vi "play_auto_id-old.vi"(8 "error in":errorcluster, 11 "Swept-Sines-Control-Settings":cluster{"u-max":sgl, "offset":sgl, "Ki":sgl}={"u-max"=1.0, "offset"=0.3, "Ki"=0.0}) -> (0 "error out":errorcluster, 1 "Is-Totally-Stable":bool)   [LabVIEW 2017]
uses:
  controls/SS_SweptSines.ctl
  controls/SS_sin_params.ctl
  controls/SS_input_data_json.ctl
  controls/fit_sos_results.ctl
  controls/auto_id_result.ctl
  controls/SOS_frf_data.ctl
  controls/SS_figures.ctl
  controls/bode_figure.ctl
  controls/logging_selection.ctl
  <vilib>/Utility/error.llb/DialogType.ctl
  <vilib>/FPGAPlugInAG/cRIO-9082/niLvFpga_Open_cRIO-9082.vi
  <vilib>/rvi/interface/common/dynamic/niFpgaDynamicAddResources.vi
  <vilib>/FPGAPlugInAG/Dynamic/niLvFpga_Reset_Dynamic.vi
  <vilib>/rvi/interface/common/niFpgaWaitOnOcc.vi
  <vilib>/Utility/error.llb/Error Cluster From Error Code.vi
  <vilib>/rvi/errors/niLvFpgaAdjustHostInterfaceError.vi
  <vilib>/FPGAPlugInAG/Dynamic/niLvFpga_Run_Dynamic.vi
  <vilib>/FPGAPlugInAG/Dynamic/niLvFpga_Close_Dynamic.vi
  <vilib>/rvi/interface/nirviOpenFPGA/nirviOpenFPGA.xnode
  FPGA Bitfiles/afmimagingcontro_FPGATargetSPARTA_SSfpgasweptsines_lpZqvyn1KNg.lvbitx
  <vilib>/rvi/interface/nirviMethod/nirviMethod.xnode
  <vilib>/rvi/interface/nirviReadWriteControl/nirviReadWriteControl.xnode
  <vilib>/rvi/interface/nirviCloseFPGA/nirviCloseFPGA.xnode
  labview/utils_lib/utils.lvlib
  NiFpgaLv.dll
  <vilib>/rvi/interface/Simulation/niFpgaSimulationCallBeginRW.vi
  <vilib>/addons/_JKI.lib/Serialization/JSON/JKI JSON Serialization.lvlib
  <vilib>/FPGAPlugInAG/Dynamic/niLvFpga_ConfigureFifo_Dynamic.vi
  <vilib>/rvi/errors/niLvFpgaMergeErrorWithErrorCode.vi
panel:
  in  "Tab Control":enum32{"Page 1", "debug"}(tab)
  in  "control-xy-to-zero":bool=TRUE
  in  "Amplitude":dbl=0.12 format="%#_13g"
  in  "ABORT":bool
  out "auto_id_result":T1
  out "fit_sos_result":T3
  in  "theta0":dbl[](array[numeric])=[0.6786, -1.9959, 0.99891, -1.996142, 0.9989]
  out "theta-fit":dbl[](array[numeric])
  out "Bode amplitude":cluster{"W":dbl[], "Magnitude":dbl[]}[](graph) caption="Magnitude Graph"
  in  "Input File (json)":path=path "Z:/afm-cs/sysID/z-axis_sines_info_quick_firstRes.json"
  in  "output-file":path=path "C:/Users/arnold/Documents/afm-cs/labview/first_res_fit.json"
  out "boolean  indicators":T4
  out "Freqs Done":i32(slide) scale=0.0..50.0
  out "number_of_freqs":i32
  out "freq_adjusted":dbl
  in  "SweptSines (in)":T5={"Log-Channel_select"=[FALSE, FALSE, FALSE, FALSE, FALSE, FALSE], "JSON Header"="", "SS-Params-Array"=[], "input_frequency_definitions"={"Amp"=0.0, "Ts"=0.0, "num_periodsMT"=[], "freqs_Hz"=[], "numAve_s"=[], "Nsamp_total"=[], "Nsettle_s"=[], "Ncollect_s"=[]}, "DAC-ADC primary 2"=0, "Channel-Names"=[], "num_chan"=0, "num-freqs"=0, "Input File (json)"=path "Z:/afm-cs/sysID/x-axis_sines_info_intsamps_quick.json"} {"DAC-ADC primary 2" items=["DAC0/ADC0", "DAC1/ADC1", "DAC2/ADC2", "DAC3/ADC3", ""]}
  out "TsTicks":u32
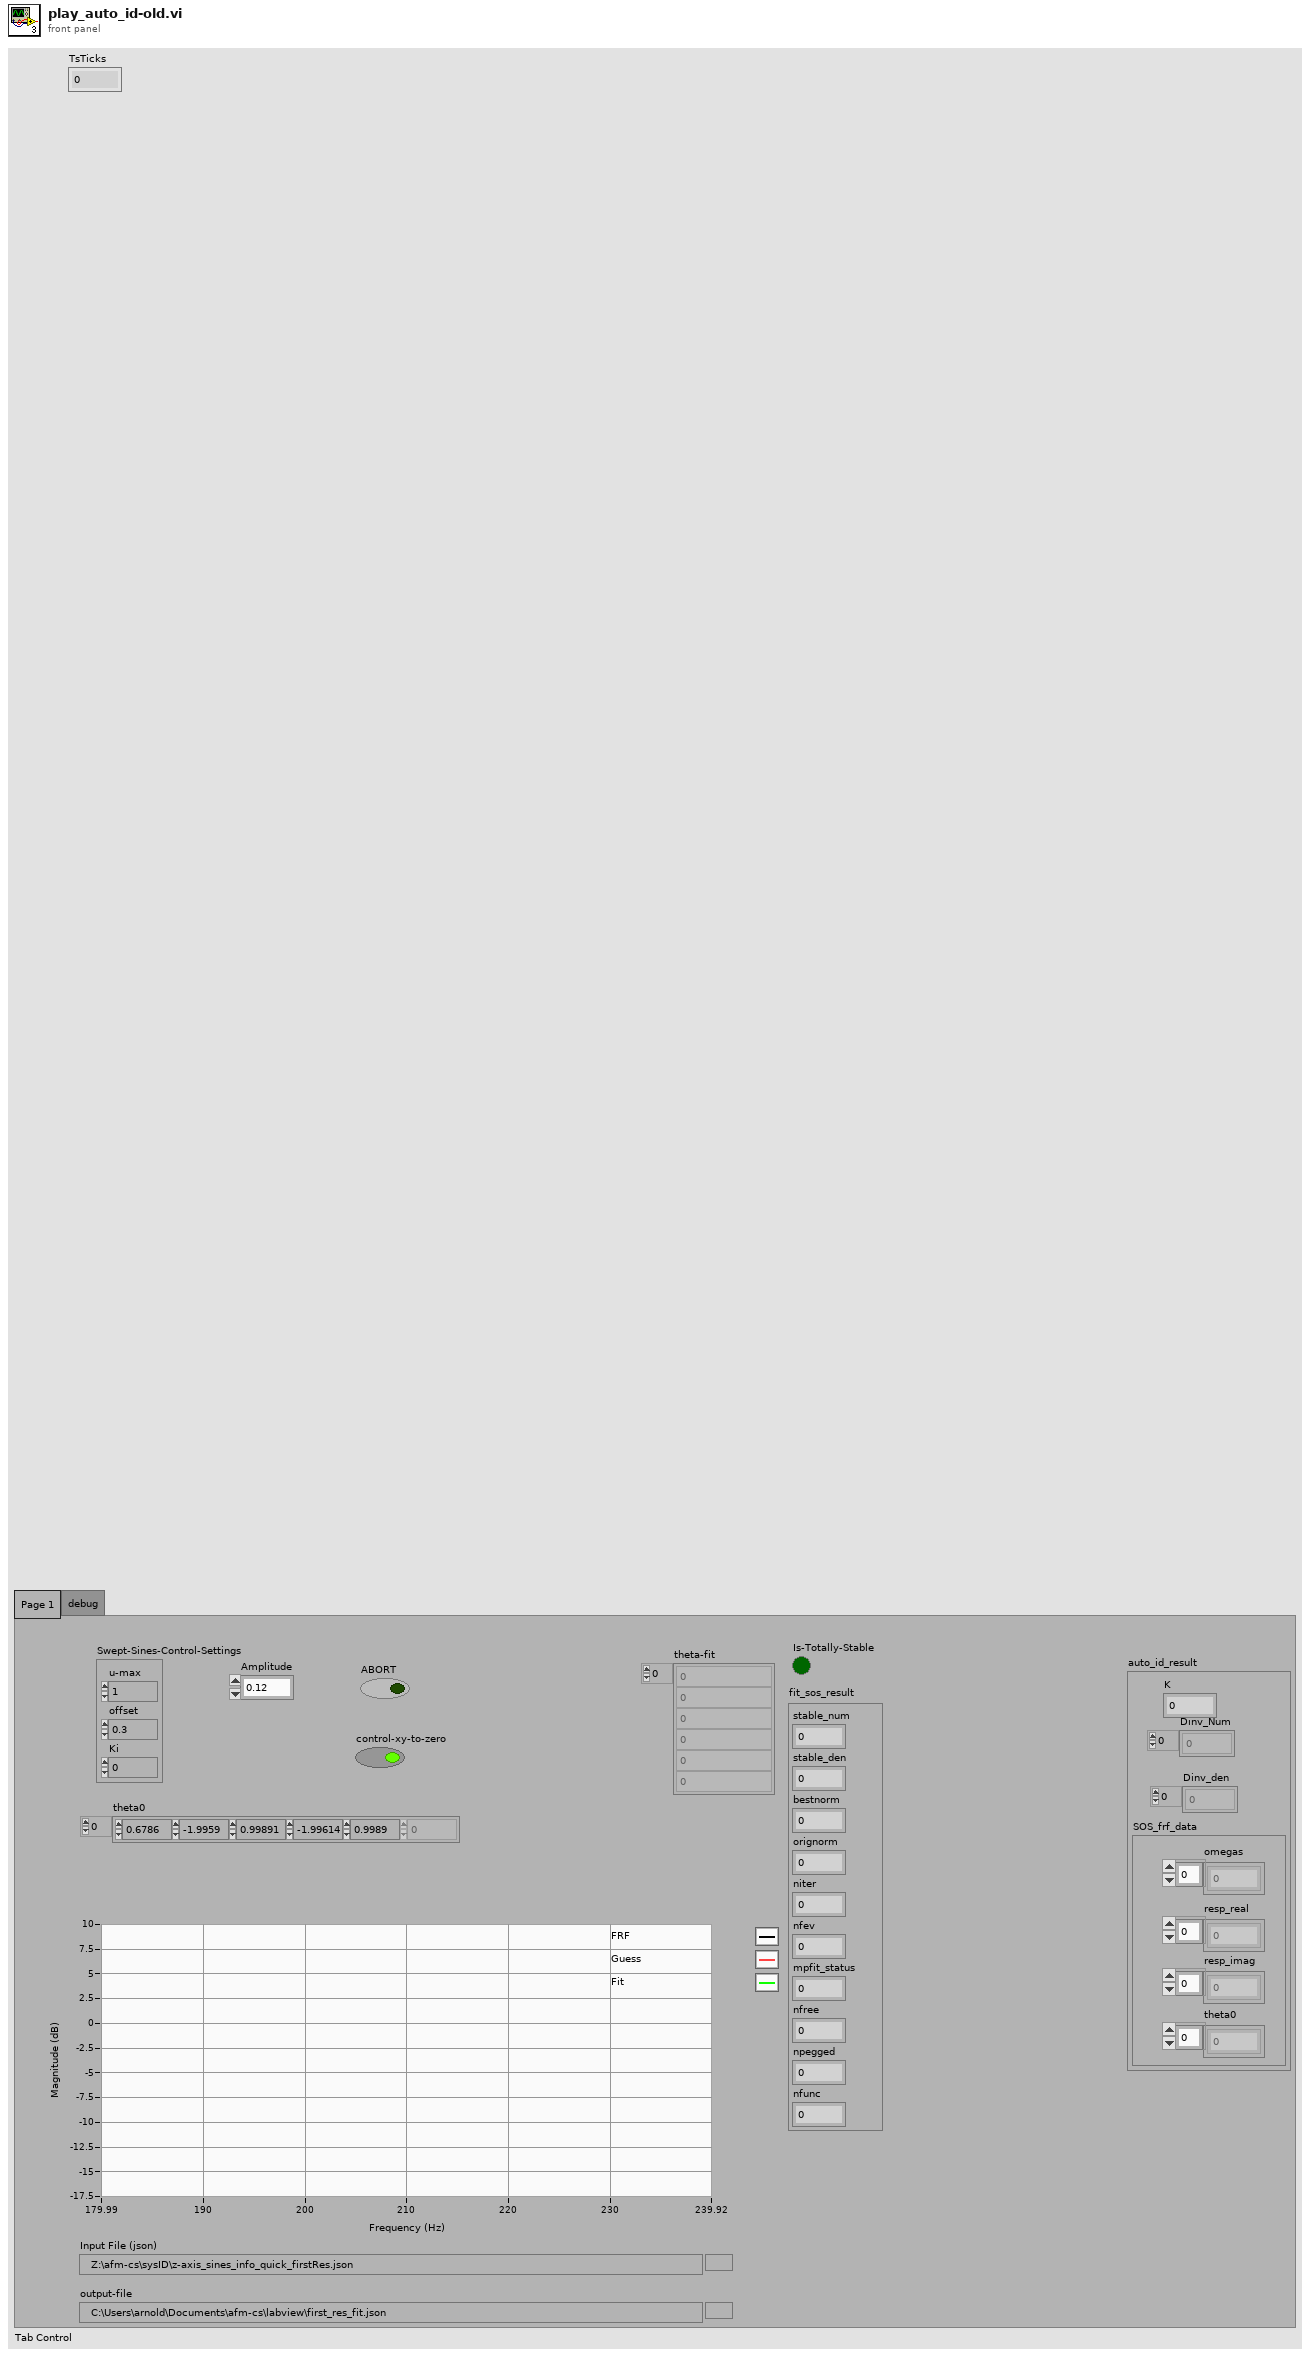
[diagram p1: front panel]
types:
  T1 = typedef "auto_id_result.ctl" = cluster{"Dinv_Num":dbl[], "SOS_frf_data":T2, "Dinv_den":dbl[], "K":dbl}
  T2 = typedef "SOS_frf_data.ctl" = cluster{"omegas":dbl[], "resp_real":dbl[], "resp_imag":dbl[], "theta0":dbl[]}
  T3 = typedef "fit_sos_results.ctl" = cluster{"stable_num":i32, "stable_den":i32, "bestnorm":dbl, "orignorm":dbl, "niter":i32, "nfev":i32, "mpfit_status":i32, "nfree":i32, "npegged":i32, "nfunc":i32}
  T4 = cluster{"unstable-z-traj":bool, "input fifo time-out":bool, "logging fifo timeout":bool, "scanning finished":bool, "unstable-x-traj":bool, "unstable-y-traj":bool, "ABORT":bool, "All Measurements Done":bool, "fpga_finished":bool, "current_scan_finished":bool}
  T5 = typedef "SS_SweptSines.ctl" = cluster{"Log-Channel_select":bool[], "JSON Header":string, "SS-Params-Array":T6[], "input_frequency_definitions":T7, "DAC-ADC primary 2":i16, "Channel-Names":string[], "num_chan":i32, "num-freqs":i32, "Input File (json)":path}
  T6 = typedef "SS_sin_params.ctl" = cluster{"freq":dbl, "num_samples":i32, "Amp":dbl, "Ts":dbl, "N_settle":u32, "Ncollect":i32, "num_periodsMT":i32, "num_averages":i32}
  T7 = typedef "SS_input_data_json.ctl" = cluster{"Amp":dbl, "Ts":dbl, "num_periodsMT":u32[], "freqs_Hz":dbl[], "numAve_s":i32[], "Nsamp_total":u32[], "Nsettle_s":u32[], "Ncollect_s":u32[]}
  T8 = typedef "logging_selection.ctl" = cluster{"Collect reference":bool, "Collect DAC control":bool, "Collect AI-0":bool, "Collect AI-1":bool, "Collect AI-2":bool, "Collect AI-3":bool}
  T9 = typedef "SS_figures.ctl" = cluster{"bode figures":T10, "Freqs Done":refnum<vi>}
  T10 = typedef "bode_figure.ctl" = cluster{"Bode phase":refnum<vi>, "Bode amplitude":refnum<vi>}
  T11 = typedef "FrdData.ctl" = cluster{"Frequency Unit":enum16{"Hz", "rad/s"}, "W":dbl[], "MagDB":dbl[], "PhaseDeg":dbl[], "Resp":cdb[], "Data-name":string}
  T12 = typedef "DialogType.ctl" = u16
  T13 = typedef "SS_experimental-data.ctl" = cluster{"sin-data-out":dbl[][], "Fourier Data":T14, "freq_adjusted?":dbl, "below-nyquist":bool}
  T14 = typedef "SS_FourierData.ctl" = cluster{"E_s":dbl[], "Fourier Coefs":cdb[], "freq-adjusted":dbl}
  T15 = enum16{"open", "replace", "create", "open or create", "replace or create", "replace or create with confirmation"}
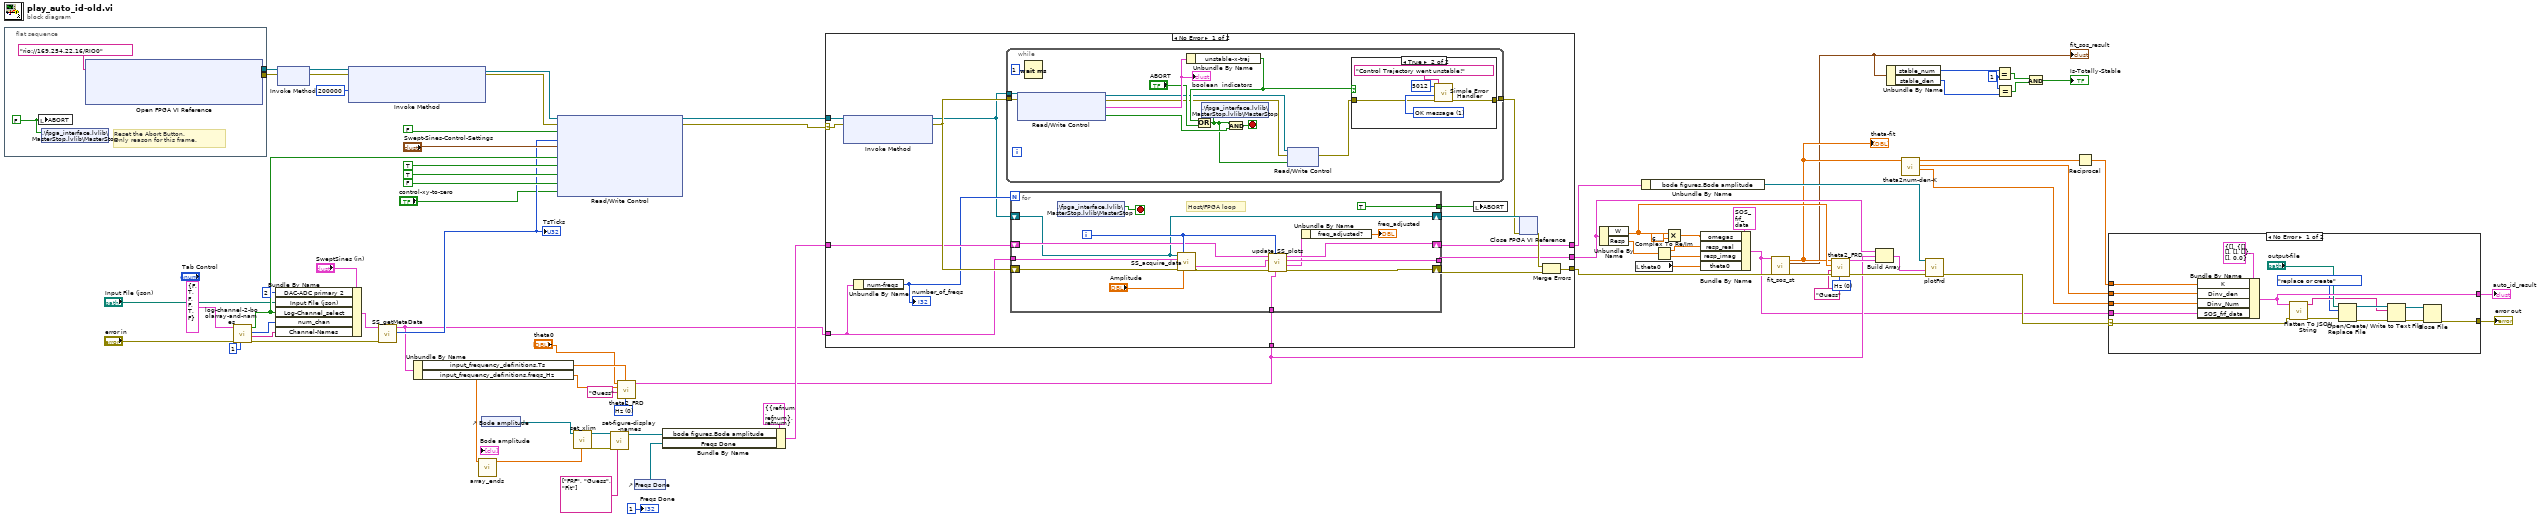
[diagram p0: block diagram]
diagram:
  w14 = 1
  w39 = u16 0 items=["Hz", "rad/s"] ("freq unit")
  w48 = u16 0 items=["Hz", "rad/s"] ("freq unit")
  n1 = flat-sequence {
    tunnel: [w81] -> w77
    tunnel: [w80] -> w76
    frame #0 {
      w79 = FALSE
      # "Reset the Abort Button.\nOnly reason for this frame."
      n2 = local write "ABORT"(w79) -> ()
      n3 = shared-variable ".\\fpga_interface.lvlib\\MasterStop.lvlib\\MasterStop"(w79) -> ()  [unwired: 1 in, 1 out]
      n4 = xnode "Open FPGA VI Reference"("resource name"=tag "rio://169.254.22.16/RIO0") -> ("FPGA VI Reference Out"=w81:refnum<k20>, "error out"=w80:errorcluster)  [unwired: 1 in]
    }
  }
  n5 = call "log-channel-2-boolarray-and-names.vi"("min_number_chan"=i16 1, "error in"="error in", "Logging selection"=T8 {"Collect reference"=FALSE, "Collect DAC control"=TRUE, "Collect AI-0"=FALSE, "Collect AI-1"=FALSE, "Collect AI-2"=TRUE, "Collect AI-3"=FALSE}) -> ("error out"=w65:errorcluster, "Channel-Names"=w63:string[], "num_chan"=w60:i32, "Log-Channel_select"=w58:bool[])  [unwired: 5 in]
  n6 = Bundle By Name(cluster="SweptSines (in)", "DAC-ADC primary 2"=i16 2, "Input File (json)"="Input File (json)", "Log-Channel_select"=w58, "num_chan"=w60, "Channel-Names"=w63) -> (w62:T5)
  n7 = xnode "Invoke Method"("FPGA VI Reference In"=w77, "error in"=w76) -> ("FPGA VI Reference Out"=w70:refnum<k20>, "error out"=w69:errorcluster)
  n8 = xnode "Invoke Method"("FPGA VI Reference In"=w70, "error in"=w69, "Requested Depth"=200000 ("requested depth")) -> ("FPGA VI Reference Out"=w75:refnum<k20>, "error out"=w71:errorcluster)  [unwired: 1 out]
  n9 = call "SS_getMetaData.vi"("error in"=w65, "SweptSines"=w62) -> ("TsTicks"=w55:u32, "SweptSines (out)"=w24:T5)  [unwired: 6 in, 1 out]
  "TsTicks" <- w55
  n10 = Unbundle By Name(w24) -> ("input_frequency_definitions.Ts"=w47:dbl, "input_frequency_definitions.freqs_Hz"=w46:dbl[])
  n11 = call "array_ends.vi"("freqs_Hz"=w46) -> ("Array"=w50:dbl[])  [unwired: 10 in]
  n12 = control-ref of="Bode amplitude"() -> (w53:refnum<vi>)
  n13 = xnode "Read/Write Control"("FPGA VI Reference In"=w75, "error in"=w71, "ABORT"=FALSE, "TsTicks"=w55, "Swept-Sines-Control-Settings"="Swept-Sines-Control-Settings", "Log-Channel_select"=w58, "Subtract y0?"=TRUE ("Subtract-origin"), "reset"=TRUE, "Close Loop?"=FALSE, "control-xy-zero"="control-xy-to-zero") -> ("FPGA VI Reference Out"=w67:refnum<k20>, "error out"=w66:errorcluster)
  n14 = call "set_xlim.vi"("xlim"=w50, "figure (in)"=w53) -> ("error out"=w51:errorcluster, "figure (out)"=w52:refnum<vi>)  [unwired: 8 in]
  n15 = call "set-figure-display-names.vi"("DisplayNames"=string[] ["FRF", "Guess", "Fit"] ("Data_names"), "error in"=w51, "figure (in)"=w52) -> ("figure (out)"=w44:refnum<vi>)  [unwired: 7 in, 1 out]
  n16 = call "theta2_FRD.vi"("freq unit"=w48, "Sampling Time (s)"=w47, "Data-name"="Guess", "freqs/omega"=w46, "theta"="theta0") -> ("FRD-model"=w25:T11)  [unwired: 5 in, 1 out]
  n17 = control-ref of="Freqs Done"() -> (w20:refnum<vi>)
  n18 = Bundle By Name(cluster=T9 {"bode figures"={"Bode phase"=refnum, "Bode amplitude"=refnum}, "Freqs Done"=refnum} ("figures"), "bode figures.Bode amplitude"=w44, "Freqs Done"=w20) -> (w43:T9)
  n19 = case shown="No Error" w66 {
    selector: w66 -> [w88 w135]
    tunnel: w67 -> [w98 _]
    tunnel: [w93 w135] -> w54
    tunnel: w24 -> [w90 _]
    tunnel: w43 -> [w91 w134]
    tunnel: [w86 w134] -> w31
    tunnel: w25 -> [w85 _]
    tunnel: [w84 _] -> w26
    frame No Error {
      n20 = xnode "Invoke Method"("FPGA VI Reference In"=w98, "error in"=w88) -> ("FPGA VI Reference Out"=w83:refnum<k20>, "error out"=w96:errorcluster)  [unwired: 1 in]
      n21 = Unbundle By Name(w90) -> ("num-freqs"=w89:i32)
      "number_of_freqs" <- w89
      n22 = while {
        tunnel: w83 -> [w110]
        tunnel: w96 -> [w109]
        tunnel: [w105] -> w92
        stop <- w101 stop-if-true
        n23 = xnode "Read/Write Control"("FPGA VI Reference In"=w110, "error in"=w109) -> ("FPGA VI Reference Out"=w104:refnum<k20>, "error out"=w103:errorcluster, "boolean  indicators"=w108:T4, "All Done"=w100:bool)
        "boolean  indicators" <- w108
        n24 = Wait (ms)(milliseconds to wait=u32 1) -> ()  [unwired: 1 out]
        n25 = Unbundle By Name(w108) -> ("unstable-x-traj"=w106:bool)
        n26 = Or(x=w106, y="ABORT") -> (x .or. y?=w99:bool)
        n27 = shared-variable ".\\fpga_interface.lvlib\\MasterStop.lvlib\\MasterStop"(w99) -> ()  [unwired: 1 in, 1 out]
        n28 = And(x=w99, y=w100) -> (x .and. y?=w101:bool)
        n29 = xnode "Read/Write Control"("FPGA VI Reference In"=w104, "error in"=w103, "ABORT"=w99) -> ("error out"=w102:errorcluster)  [unwired: 1 out]
        n30 = case shown="True" w106 {
          tunnel: w102 -> [w112 w114]
          tunnel: [w112 w113] -> w105
          frame False {
          }
          frame True {
            w117 = T12 1 items=["no dialog", "OK message", "continue or stop message", "OK message + warnings", "continue/stop + warnings"] ("type of dialog (OK msg:1)")
            n31 = call <vilib>:"Simple Error Handler.vi"("error code (no error:0)"=5012, "error source (\" \")"="Control Trajectory went unstable!" ("error source (\" \")"), "type of dialog (OK msg:1)"=w117, "error in (no error)"=w114) -> ("error out"=w113:errorcluster)  [unwired: 1 in, 4 out]
          }
        }
      }
      n32 = for {
        N: w89 -> [_]
        shift-right: [w123] -> w86
        shift-left: w91 -> [w122]
        tunnel: [TRUE] -> w95
        shift-right: [w129] -> w87
        shift-left: w96 -> [w131]
        tunnel: w90 -> [w130]
        tunnel: [w124] -> w84
        tunnel: w85 -> [w120]
        shift-right: [w118] -> w97
        shift-left: w83 -> [w118]
        i -> [w127]
        stop <- w119 stop-if-true
        # "Host/FPGA loop"
        n33 = shared-variable ".\\fpga_interface.lvlib\\MasterStop.lvlib\\MasterStop"() -> (w119:bool)  [unwired: 1 in, 1 out]
        n34 = call "SS_acquire_data.vi"("Type"=w118, "idx"=w127, "SweptSines (in)"=w130, "error in"=w131, "Signal Amplitude (V)"="Amplitude") -> ("experiment-data"=w126:T13, "error IO"=w125:errorcluster)  [unwired: 7 in, 2 out]
        n35 = call "update_SS_plots.vi"("other-frd"=w120, "freqs-iter"=w127, "error in (no error)"=w125, "experiment-data"=w126, "figures-in"=w122) -> ("error out"=w129:errorcluster, "experiment-data (out)"=w121:T13, "FRD-out"=w124:T11, "figures-out"=w123:T9)  [unwired: 3 in]
        n36 = Unbundle By Name(w121) -> ("freq_adjusted?"=→"freq_adjusted":dbl)
      }
      n37 = local write "ABORT"(w95) -> ()
      n38 = xnode "Close FPGA VI Reference"("FPGA VI Reference In"=w97, "error in"=w92) -> ("error out"=w94:errorcluster)
      n39 = Merge Errors(w94, w87) -> (w93:errorcluster)
    }
    frame Error {
    }
  }
  n40 = Unbundle By Name(w26) -> ("W"=w19:dbl[], "Resp"=w33:cdb[])
  n41 = local read "theta0"() -> (w32:dbl[])
  n42 = Unbundle By Name(w31) -> ("bode figures.Bode amplitude"=w27:refnum<vi>)
  n43 = Complex To Re/Im(x + iy=w33) -> (x=w35:dbl[], y=w34:dbl[])
  n44 = Multiply(x=w19, y=6.283185307179586) -> (x*y=w37:dbl[])
  n45 = Bundle By Name(cluster=T2 {"omegas"=[1006.674891, 1016.262272, 1025.849652, 1035.437033, 1045.024413, 1054.611794, 1064.199174, 1073.786548, 1083.373929, 1092.961309, 1102.54869, 1112.13607, 1121.723451, 1131.310831, 1140.898212, 1150.485592, 1160.072973, 1169.660354, 1179.247728, 1188.835108, 1198.422489, 1208.009869, 1217.59725, 1227.18463, 1236.772011, 1246.359391, 1255.946772, 1265.534152, 1275.121533, 1284.708907, 1294.296288, 1303.883668, 1313.471049, 1323.058429, 1332.64581, 1342.23319, 1351.820571, 1361.407951, 1370.995332, 1380.582706, 1390.170086, 1399.757467, 1409.344847, 1418.932228, 1428.519609, 1438.106989, 1447.69437, 1457.28175, 1466.869131, 1476.456511, 1486.043885, 1495.631266, 1505.218646, 1514.806027, 1524.393407, 1533.980788, 1543.568168, 1553.155549, 1562.742929, 1572.33031, 1581.91769, 1591.505065, 1601.092445, 1610.679826, 1620.267206, 1629.854587, 1639.441967, 1649.029348, 1658.616728], "resp_real"=[0.6710936201, 0.6732167298, 0.6736550301, 0.6739624194, 0.6764113406, 0.6760996891, 0.6752809587, 0.67695858, 0.6764911126, 0.6818501379, 0.6804259731, 0.6777421689, 0.683602427, 0.6839502494, 0.6873055899, 0.6871681129, 0.6836241729, 0.6933718335, 0.6965190689, 0.7011525702, 0.7041006273, 0.7087951209, 0.7138881005, 0.7230810664, 0.7347158563, 0.743593779, 0.7581554602, 0.7740064901, 0.7983882262, 0.8168799192, 0.8500537495, 0.885993569, 0.8534751304, 0.6135298299, 0.1963078728, 0.06997493602, 0.2143720387, 0.3262401307, 0.3874363268, 0.4244315327, 0.4518076771, 0.4783094111, 0.4942330365, 0.5078067569, 0.5183774173, 0.5254372068, 0.5346584888, 0.5422376, 0.5476692529, 0.546204086, 0.5501300272, 0.5526801006, 0.557631838, 0.5639162136, 0.5601299408, 0.5627301292, 0.5646599194, 0.5678509651, 0.5674161925, 0.5676099823, 0.5703128211, 0.5717199117, 0.5717616028, 0.5714305364, 0.5706488864, 0.574491682, 0.5720673373, 0.5722619255, 0.5727540208], "resp_imag"=[0.1828230252, 0.185702312, 0.1893108783, 0.1927179342, 0.1939516982, 0.1991804891, 0.1996588255, 0.1997489381, 0.2009184192, 0.2058333084, 0.205968755, 0.2071290225, 0.2120033665, 0.2140896781, 0.2197333799, 0.2218060221, 0.2270970718, 0.2243543787, 0.2282290931, 0.2349554807, 0.2362899955, 0.2386023634, 0.2479762836, 0.2514213949, 0.2589829258, 0.2690734156, 0.2817668466, 0.3075000844, 0.3292949756, 0.3581777586, 0.418098085, 0.518537997, 0.7274335428, 0.9954410219, 0.8283414758, 0.4651799029, 0.2632646215, 0.2204933474, 0.2100370796, 0.215817828, 0.2094899805, 0.2041701149, 0.2090161752, 0.2122336611, 0.2144513636, 0.2154505064, 0.2184072105, 0.2207006189, 0.2264320741, 0.2319746485, 0.2352243002, 0.2359211056, 0.2344839067, 0.234200787, 0.2350554818, 0.2419460399, 0.2451480379, 0.2422561944, 0.2450402058, 0.2520603413, 0.2526693987, 0.2530329194, 0.2523935129, 0.2570623818, 0.2576871444, 0.2563998974, 0.259830217, 0.2610581842, 0.2647075477], "theta0"=[0.6786, -1.9959, 0.99891, -1.996142, 0.9989]} ("SOS-frf_data"), "omegas"=w37, "resp_real"=w35, "resp_imag"=w34, "theta0"=w32) -> (w7:T2)
  n46 = call "fit_sos_st.vi"("frf_data"=w7, "error in (no error)"=w54) -> ("theta"=w18:dbl[], "fit_sos_result"=w17:T3, "error out"=w41:errorcluster)  [unwired: 23 in]
  "fit_sos_result" <- w17
  "theta-fit" <- w18
  n47 = call "theta2_FRD.vi"("freq unit"=w39, "error in (no error)"=w41, "Data-name"="Guess", "freqs/omega"=w19, "theta"=w18) -> ("error out"=w28:errorcluster, "FRD-model"=w30:T11)  [unwired: 5 in]
  n48 = Build Array(w26, w25, w30) -> (w29:T11[])
  n49 = Unbundle By Name(w17) -> ("stable_num"=w16:i32, "stable_den"=w15:i32)
  n50 = call "theta2num-den-K.vi"("theta"=w18) -> ("Den"=w3:dbl[], "Num"=w8:dbl[], "K"=w2:dbl)  [unwired: 8 in]
  n51 = call "plotFrd.vi"("error in (no error)"=w28, "FRD-array"=w29, "Magnitude Graph Reference in"=w27) -> ("error out"=w9:errorcluster)  [unwired: 6 in, 2 out]
  n52 = Equal?(x=w16, y=w14) -> (x = y?=w12:bool)
  n53 = Equal?(x=w14, y=w15) -> (x = y?=w13:bool)
  n54 = And(x=w12, y=w13) -> (x .and. y?=→"Is-Totally-Stable":bool)
  n55 = Reciprocal(x=w2) -> (1/x=w1:dbl)
  n56 = case shown="No Error" w9 {
    selector: w9 -> [w147 w152]
    tunnel: w3 -> [w150 _]
    tunnel: w8 -> [w149 _]
    tunnel: w7 -> [w148 _]
    tunnel: [w139 w152] -> w5
    tunnel: [w146 _] -> w6
    tunnel: w1 -> [w136 _]
    frame No Error {
      n57 = Bundle By Name(cluster=T1 {"Dinv_Num"=[], "SOS_frf_data"={"omegas"=[], "resp_real"=[], "resp_imag"=[], "theta0"=[]}, "Dinv_den"=[], "K"=0.0} ("auto_id_result 2"), "K"=w136, "Dinv_den"=w149, "Dinv_Num"=w150, "SOS_frf_data"=w148) -> (w146:T1)
      n58 = call <vilib>:"Flatten To JSON String.vi"("error in (no error)"=w147, "Variant"=w146) -> ("error out"=w144:errorcluster, "JSON String"=w141:string)  [unwired: 8 in]
      n59 = Open/Create/Replace File(file path (use dialog)="output-file", error in=w144, operation (0:open)=T15."replace or create") -> (refnum out=w145:refnum<file>, error out=w143:errorcluster)  [unwired: 3 in, 1 out]
      n60 = Write to Text File(file (use dialog)=w145, text=w141, error in=w143) -> (refnum out=w138:refnum<file>, error out=w140:errorcluster)  [unwired: 1 in, 1 out]
      n61 = Close File(refnum=w138, error in=w140) -> (error out=w139:errorcluster)  [unwired: 1 out]
    }
    frame Error {
    }
  }
  "error out" <- w5
  "auto_id_result" <- w6
  "Freqs Done" <- 1 ("Freqs Done")
